vi "Spin pumping.vi"() -> ()   [LabVIEW 2020]
uses:
  <vilib>/Utility/file.llb/Write Delimited Spreadsheet (DBL).vi
panel:
  out "Multicolumn Listbox 2":i32(listbox)
  out "Current Measurement Phase":cluster{dbl[], dbl[]}(graph)
  out "Current Measurement Amplitude":cluster{dbl[], dbl[]}(graph)
  out "Last Measurement Phase":cluster{dbl[], dbl[]}(graph)
  out "Last Measurement Amplitude":cluster{dbl[], dbl[]}(graph)
  in  "SR830 GPIB Addr":dbl
  in  "AM Depth (%)":dbl
  in  "AM Freq (Hz)":dbl
  in  "Multicolumn Listbox":i32(listbox)
  in  "# of pt":dbl
  in  "Kepco Max I":dbl
  in  "Kepco GPIB Addr":dbl
  in  "SMB 100a GPIB Addr":dbl
  in  "Model 7010 GPIB Addr":dbl
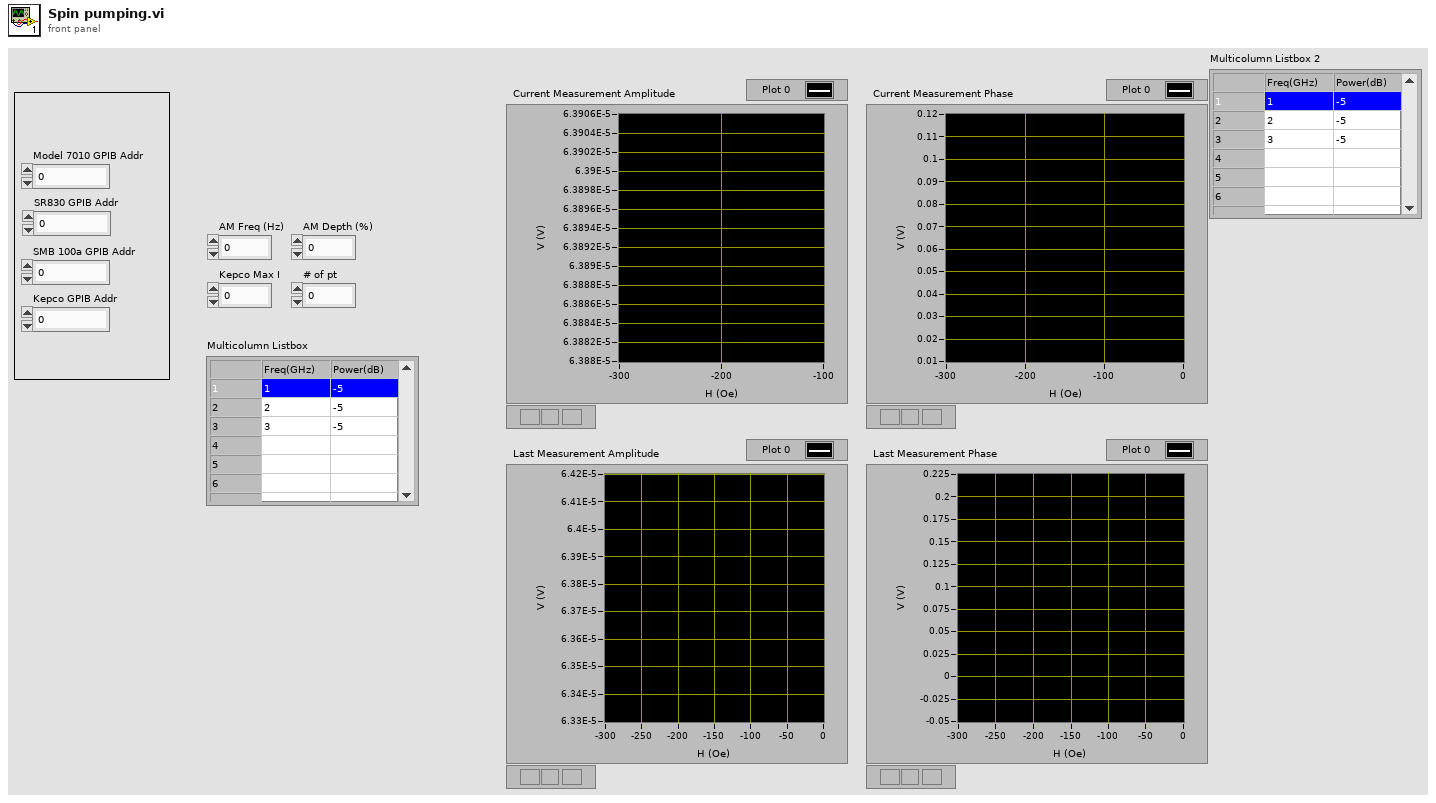
[diagram p1: front panel]
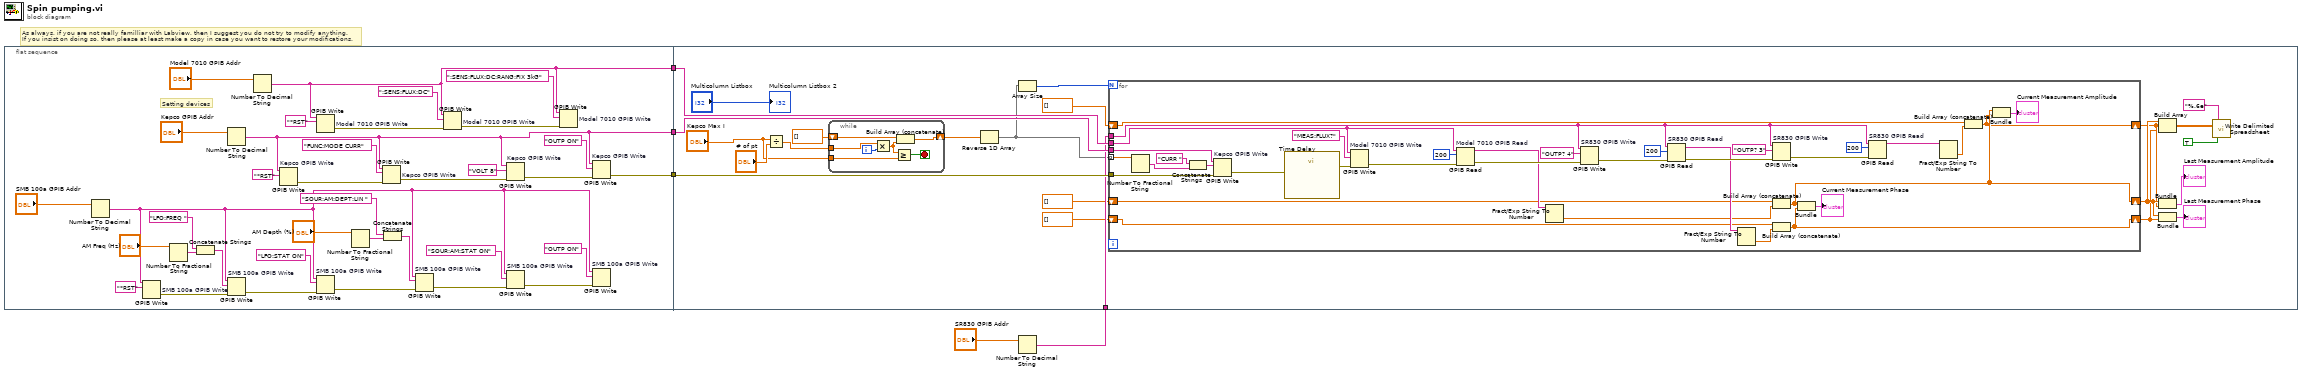
[diagram p0: block diagram]
diagram:
  # "As always, if you are not really familliar with Labview, then I suggest you do not try to modify anything.\nIf you insist on doing so, then please at least make a copy in case you want to restore your modifications."
  n1 = flat-sequence {
    tunnel: [w11] -> w3
    tunnel: [w10] -> w4
    tunnel: [w9] -> w5
    tunnel: w1 -> [w55]
    tunnel: w5 -> [w58]
    tunnel: w4 -> [w56]
    tunnel: w3 -> [w57]
    frame #0 {
      # "Setting devices"
      n2 = Number To Decimal String(number="SMB 100a GPIB Addr") -> (decimal integer string=w7:string)  [unwired: 1 in]
      n3 = GPIB Write "SMB 100a GPIB Write"(0:w7, 1:"*RST" ("data")) -> (6:w28:errorcluster)  [unwired: 3 in, 1 out]
      n4 = Number To Fractional String(number="AM Freq (Hz)") -> (F-format string=w31:string)  [unwired: 3 in]
      n5 = Concatenate Strings("LFO:FREQ " ("string"), w31) -> (w29:string)
      n6 = Number To Decimal String(number="Kepco GPIB Addr") -> (decimal integer string=w9:string)  [unwired: 1 in]
      n7 = GPIB Write "SMB 100a GPIB Write"(0:w7, 1:w29, 3:w28) -> (6:w27:errorcluster)  [unwired: 2 in, 1 out]
      n8 = Number To Decimal String(number="Model 7010 GPIB Addr") -> (decimal integer string=w10:string)  [unwired: 1 in]
      n9 = GPIB Write "Kepco GPIB Write"(0:w9, 1:"*RST" ("data")) -> (6:w38:errorcluster)  [unwired: 3 in, 1 out]
      n10 = GPIB Write "Model 7010 GPIB Write"(0:w10, 1:"*RST" ("data")) -> (6:w18:errorcluster)  [unwired: 3 in, 1 out]
      n11 = GPIB Write "SMB 100a GPIB Write"(0:w7, 1:"LFO:STAT ON" ("data"), 3:w27) -> (6:w24:errorcluster)  [unwired: 2 in, 1 out]
      n12 = Number To Fractional String(number="AM Depth (%)") -> (F-format string=w23:string)  [unwired: 3 in]
      n13 = GPIB Write "Kepco GPIB Write"(0:w9, 1:"FUNC:MODE CURR" ("data"), 3:w38) -> (6:w36:errorcluster)  [unwired: 2 in, 1 out]
      n14 = Concatenate Strings("SOUR:AM:DEPT:LIN " ("string"), w23) -> (w22:string)
      n15 = GPIB Write "SMB 100a GPIB Write"(0:w7, 1:w22, 3:w24) -> (6:w20:errorcluster)  [unwired: 2 in, 1 out]
      n16 = GPIB Write "Model 7010 GPIB Write"(0:w10, 1:":SENS:FLUX:DC" ("data"), 3:w18) -> (6:w16:errorcluster)  [unwired: 2 in, 1 out]
      n17 = GPIB Write "Kepco GPIB Write"(0:w9, 1:"VOLT 8" ("data"), 3:w36) -> (6:w34:errorcluster)  [unwired: 2 in, 1 out]
      n18 = GPIB Write "SMB 100a GPIB Write"(0:w7, 1:"SOUR:AM:STAT ON" ("data"), 3:w20) -> (6:w8:errorcluster)  [unwired: 2 in, 1 out]
      n19 = GPIB Write "Model 7010 GPIB Write"(0:w10, 1:":SENS:FLUX:DC:RANG:FIX 3kG" ("data"), 3:w16) -> ()  [unwired: 2 in, 2 out]
      n20 = GPIB Write "Kepco GPIB Write"(0:w9, 1:"OUTP ON" ("data"), 3:w34) -> (6:w11:errorcluster)  [unwired: 2 in, 1 out]
      n21 = GPIB Write "SMB 100a GPIB Write"(0:w7, 1:"OUTP ON" ("data"), 3:w8) -> ()  [unwired: 2 in, 2 out]
    }
    frame #1 {
      n22 = Divide(x="Kepco Max I", y="# of pt") -> (x/y=w61:dbl)
      n23 = while {
        tunnel: w61 -> [w105]
        shift-right: [w104] -> w59
        shift-left: dbl[] [] -> [w103]
        tunnel: "Kepco Max I" -> [w100]
        i -> [w106]
        stop <- w102 stop-if-true
        n24 = Multiply(x=w105, y=w106) -> (x*y=w101:dbl)
        n25 = Greater Or Equal?(x=w101, y=w100) -> (x >= y?=w102:bool)
        n26 = Build Array (concatenate)(w103, w101) -> (w104:dbl[])
      }
      n27 = Reverse 1D Array(array=w59) -> (reversed array=w46:dbl[])
      n28 = Array Size(array=w46) -> (size(s)=w45:i32)
      n29 = for {
        N: w45 -> [_]
        tunnel: w46 -> [w98] mode=indexing
        tunnel: w58 -> [w95]
        tunnel: w57 -> [w94]
        tunnel: w56 -> [w78]
        tunnel: w55 -> [w86]
        shift-right: [w71] -> w48
        shift-left: dbl[] [] -> [w83]
        shift-right: [w72] -> w49
        shift-left: dbl[] [] -> [w80]
        shift-right: [w73] -> w51
        shift-left: dbl[] [] -> [w74]
        n30 = Number To Fractional String(number=w98) -> (F-format string=w97:string)  [unwired: 3 in]
        n31 = Concatenate Strings("CURR ", w97) -> (w96:string)
        n32 = GPIB Write "Kepco GPIB Write"(0:w95, 1:w96, 3:w94) -> (6:w93:errorcluster)  [unwired: 2 in, 1 out]
        n33 = call "Time Delay"("error in (no error)"=w93) -> ("error out"=w92:errorcluster)  [unwired: 10 in]
        n34 = GPIB Write "Model 7010 GPIB Write"(0:w78, 1:"MEAS:FLUX?" ("data"), 3:w92) -> (6:w77:errorcluster)  [unwired: 2 in, 1 out]
        n35 = GPIB Read "Model 7010 GPIB Read"(0:w78, 1:200 ("byte count"), 3:w77) -> (5:w75:string, 7:w76:errorcluster)  [unwired: 2 in, 1 out]
        n36 = Fract/Exp String To Number(string=w75) -> (number=w79:dbl)  [unwired: 3 in, 1 out]
        n37 = GPIB Write "SR830 GPIB Write"(0:w86, 1:"OUTP? 4" ("data"), 3:w76) -> (6:w89:errorcluster)  [unwired: 2 in, 1 out]
        n38 = GPIB Read "SR830 GPIB Read"(0:w86, 1:200 ("byte count"), 3:w89) -> (5:w85:string, 7:w88:errorcluster)  [unwired: 2 in, 1 out]
        n39 = Fract/Exp String To Number(string=w85) -> (number=w84:dbl)  [unwired: 3 in, 1 out]
        n40 = GPIB Write "SR830 GPIB Write"(0:w86, 1:"OUTP? 3" ("data"), 3:w88) -> (6:w87:errorcluster)  [unwired: 2 in, 1 out]
        n41 = Build Array (concatenate)(w74, w79) -> (w73:dbl[])
        n42 = Build Array (concatenate)(w83, w84) -> (w71:dbl[])
        n43 = Bundle(w73, w71) -> (→"Current Measurement Phase":cluster{dbl[], dbl[]})  [unwired: 1 in]
        n44 = GPIB Read "SR830 GPIB Read"(0:w86, 1:200 ("byte count"), 3:w87) -> (5:w81:string)  [unwired: 2 in, 2 out]
        n45 = Fract/Exp String To Number(string=w81) -> (number=w82:dbl)  [unwired: 3 in, 1 out]
        n46 = Build Array (concatenate)(w80, w82) -> (w72:dbl[])
        n47 = Bundle(w73, w72) -> (→"Current Measurement Amplitude":cluster{dbl[], dbl[]})  [unwired: 1 in]
      }
      n48 = Build Array(w51, w49, w48) -> (w50:dbl[][])
      n49 = Bundle(w51, w49) -> (→"Last Measurement Amplitude":cluster{dbl[], dbl[]})  [unwired: 1 in]
      n50 = Bundle(w51, w48) -> (→"Last Measurement Phase":cluster{dbl[], dbl[]})  [unwired: 1 in]
      n51 = call-poly <vilib>:"Write Delimited Spreadsheet.vi"("format (%.3f)"="%.6e", "2D data"=w50, "transpose? (no:F)"=TRUE) -> ()  [unwired: 11 in, 2 out]
      "Multicolumn Listbox 2" <- "Multicolumn Listbox"
    }
  }
  n52 = Number To Decimal String(number="SR830 GPIB Addr") -> (decimal integer string=w1:string)  [unwired: 1 in]
